vi "analog_input_diagnostics.vi"(9 "Reset Move Fault":bool, 10 "Voltage":dbl, 11 "IDG Const":T1) -> (1 "Delta":dbl, 2 "Integrator":u32, 3 "IDG State":T2=enum."fault_high")   [LabVIEW 2011]
uses:
  idg_trust_t.ctl
  gun/gun_idg_const.ctl
panel:
  # "Analog Input Diagnostics allows us to diagnose common analog input problems"
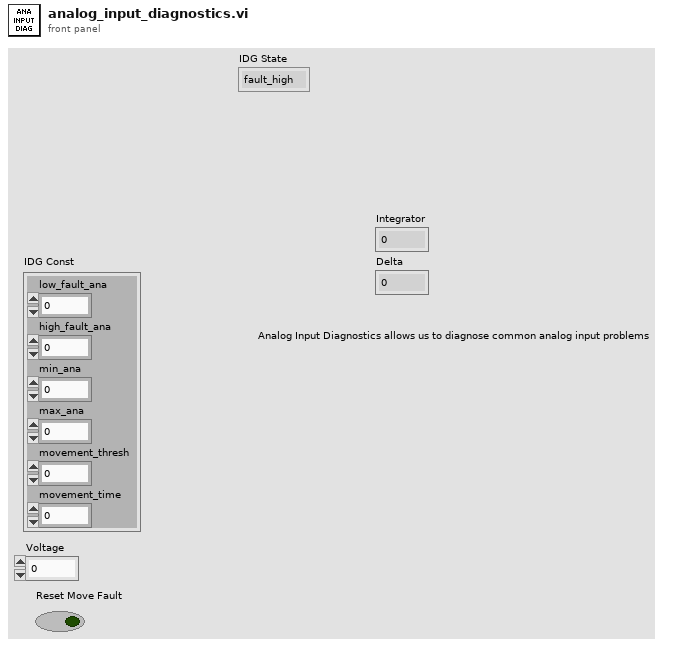
[diagram p1: front panel]
types:
  T1 = typedef "gun_idg_const.ctl" = cluster{"low_fault_ana":dbl, "high_fault_ana":dbl, "min_ana":dbl, "max_ana":dbl, "movement_thresh":dbl, "movement_time":dbl}
  T2 = typedef "idg_trust_t.ctl" = enum16{"fault_move", "fault_high", "fault_low", "out_high", "out_low", "trust"}
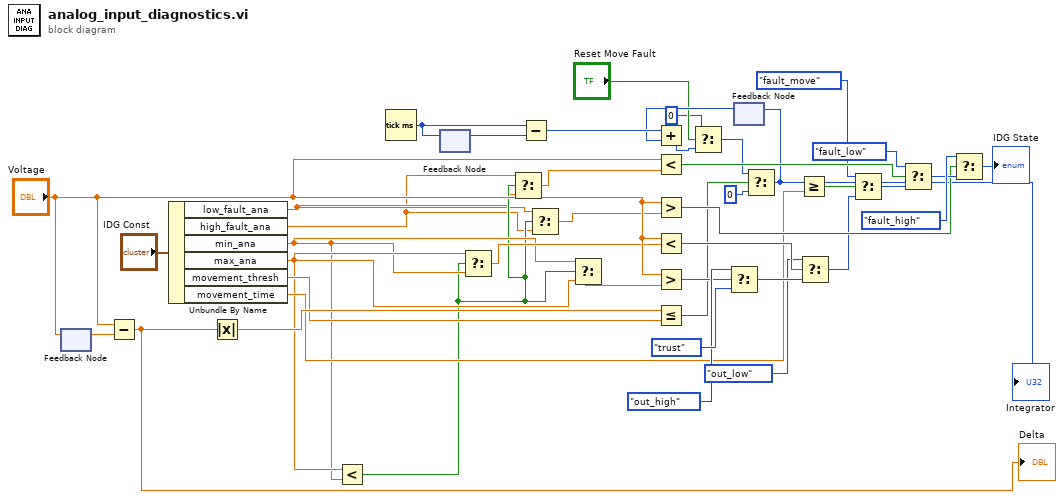
[diagram p0: block diagram]
diagram:
  n1 = feedback-in #1("Voltage") -> ()
  n2 = feedback #1() -> (w31:dbl)  [unwired: 1 in]
  n3 = Subtract(x="Voltage", y=w31) -> (x-y=w29:dbl)
  "Delta" <- w29
  n4 = Unbundle By Name("IDG Const") -> ("low_fault_ana"=w7:dbl, "high_fault_ana"=w5:dbl, "min_ana"=w10:dbl, "max_ana"=w12:dbl, "movement_thresh"=w27:dbl, "movement_time"=w19:dbl)
  n5 = Absolute Value(x=w29) -> (abs(x)=w28:dbl)
  n6 = Less?(x=w12, y=w10) -> (x < y?=w8:bool)
  n7 = Tick Count (ms)() -> (millisecond timer value=w25:u32)
  n8 = feedback-in #2(w25) -> ()
  n9 = feedback #2() -> (w26:u32)  [unwired: 1 in]
  n10 = Select(t=w12, s=w8, f=w10) -> (s? t:f=w13:dbl)
  n11 = Select(t=w5, s=w8, f=w7) -> (s? t:f=w6:dbl)
  n12 = Subtract(x=w25, y=w26) -> (x-y=w23:u32)
  n13 = Select(t=w7, s=w8, f=w5) -> (s? t:f=w9:dbl)
  n14 = Select(t=w10, s=w8, f=w12) -> (s? t:f=w11:dbl)
  n15 = Less?(x="Voltage", y=w6) -> (x < y?=w33:bool)
  n16 = Greater?(x="Voltage", y=w9) -> (0:w35:bool)
  n17 = Less?(x="Voltage", y=w13) -> (x < y?=w39:bool)
  n18 = Greater?(x="Voltage", y=w11) -> (0:w40:bool)
  n19 = Less Or Equal?(x=w28, y=w27) -> (x <= y?=w24:bool)
  n20 = Select(t=idg_trust_t."out_high", s=w40, f=idg_trust_t."trust" ("t")) -> (s? t:f=w41:T2)
  n21 = feedback #3() -> (w22:u32)  [unwired: 1 in]
  n22 = Add(x=w23, y=w22) -> (x+y=w3:u32)
  n23 = Select(t=u32 0, s="Reset Move Fault", f=w3) -> (s? t:f=w2:u32)
  n24 = Select(t=w2, s=w24, f=u32 0) -> (s? t:f=w20:u32)
  "Integrator" <- w20
  n25 = feedback-in #3(w20) -> ()
  n26 = Greater Or Equal?(x=w20, y=w19) -> (x >= y?=w18:bool)
  n27 = Select(t=idg_trust_t."out_low", s=w39, f=w41) -> (s? t:f=w16:T2)
  n28 = Select(t=idg_trust_t."fault_move", s=w18, f=w16) -> (s? t:f=w15:T2)
  n29 = Select(t=idg_trust_t."fault_low", s=w33, f=w15) -> (s? t:f=w36:T2)
  n30 = Select(t=idg_trust_t."fault_high", s=w35, f=w36) -> (s? t:f=→"IDG State":T2)
